vi "generateVang.vi"(5 "Vang_limit":dbl=4.0, 7 "PID Gains Angle":T1={"proportional gain (Kc)"=5.0, "integral time (Ti, min)"=0.0, "derivative time (Td, min)"=-2.0}, 8 "error in (no error)":errorcluster, 9 "Dest":dbl[](array[numeric])=[4500.0, 3000.0] format="%#_13g", 10 "Robot":refnum<class "Robot.lvclass">, 11 "Game in":refnum<class "Game.lvclass">) -> (0 "error out":errorcluster, 2 "Vang":dbl, 3 "Game out":refnum<class "Game.lvclass">)   [LabVIEW 2020, in "Game.lvclass"]
uses:
  Game.lvclass
  Robot_class/Robot.lvclass
  C:/RoboIME/SSL_AI/Object_class/Object.lvclass
  Object_class/Object.lvclass/Object.ctl
  Robot_class/Robot.lvclass/Robot.ctl
  <vilib>/Analysis/coordinate.llb/Wrap Angle (scalar).vi
  Object_class/Read x.vi
  Object_class/Read y.vi
  Robot_class/Read orientation.vi
  <vilib>/Analysis/NI_AAL_Angle.lvlib
panel:
  in  "Reinitialize":bool
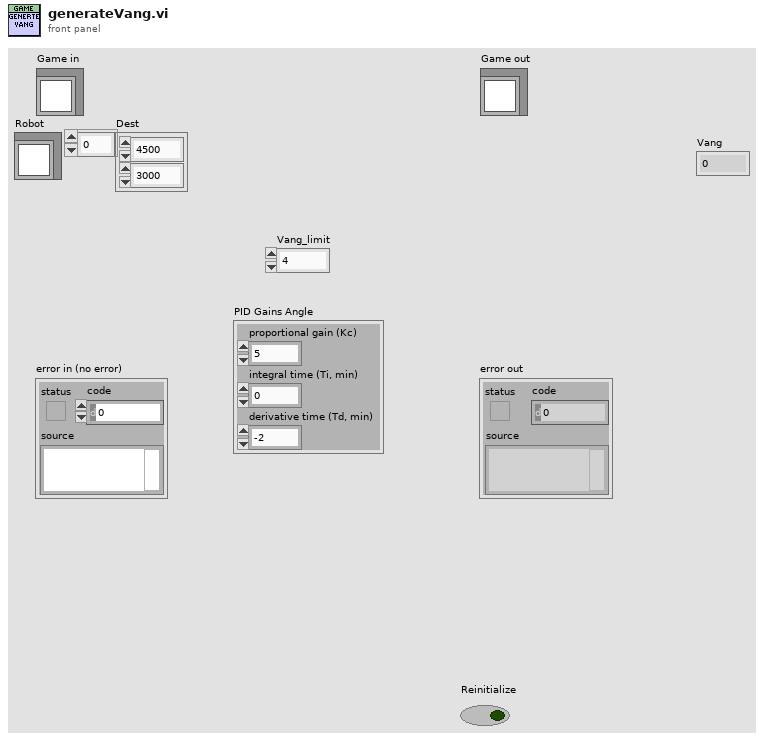
[diagram p1: front panel]
types:
  T1 = cluster{"proportional gain (Kc)":dbl, "integral time (Ti, min)":dbl, "derivative time (Td, min)":dbl}
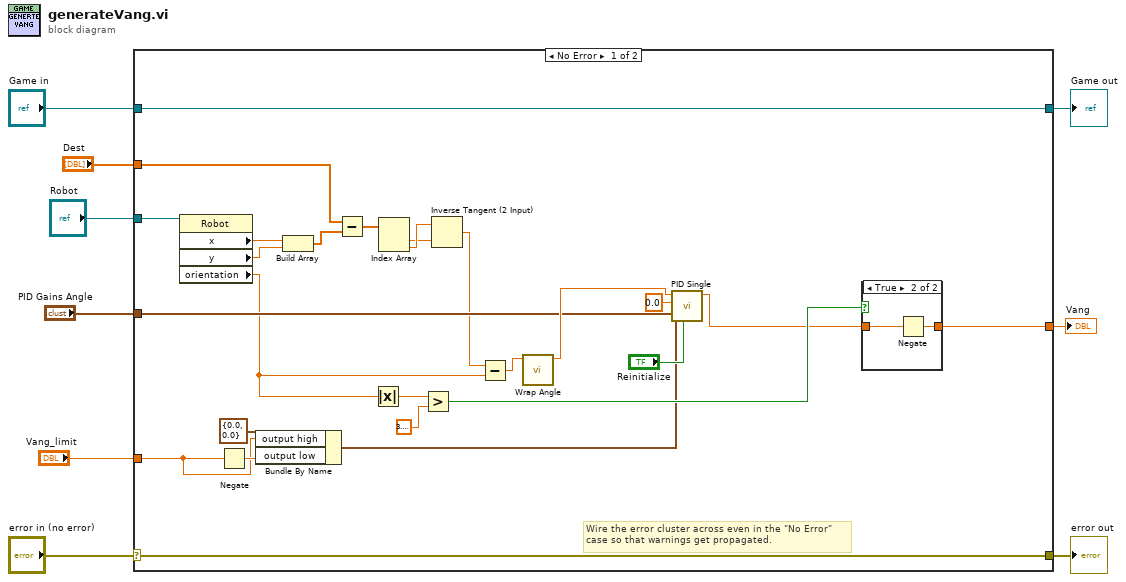
[diagram p0: block diagram]
diagram:
  n1 = case shown="No Error" "error in (no error)" {
    selector: "error in (no error)" -> [w34 w40]
    tunnel: [w34 w40] -> w8
    tunnel: [w35 w39] -> w6
    tunnel: "Game in" -> [w35 w39]
    tunnel: [w22 _] -> w5
    tunnel: "Vang_limit" -> [w21 _]
    tunnel: "PID Gains Angle" -> [w20 _]
    tunnel: "Robot" -> [w19 _]
    tunnel: "Dest" -> [w15 _]
    frame No Error {
      # "Wire the error cluster across even in the \"No Error\"\ncase so that warnings get propagated."
      n2 = property class="Robot"(reference=w19) -> ("x"=w17:dbl, "y"=w16:dbl, "orientation"=w18:dbl)  [unwired: 1 in, 2 out]
      n3 = Negate(x=w21) -> (-x=w24:dbl)
      n4 = Bundle By Name(cluster=cluster{"output high":dbl, "output low":dbl} {"output high"=0.0, "output low"=0.0}, "output high"=w21, "output low"=w24) -> (w23:cluster{"output high":dbl, "output low":dbl})
      n5 = Build Array(w17, w16) -> (w14:dbl[])
      n6 = Subtract(x=w15, y=w14) -> (x-y=w13:dbl[])
      n7 = Absolute Value(x=w18) -> (abs(x)=w33:dbl)
      n8 = Index Array(array=w13) -> (element #1=w11:dbl, element #2=w12:dbl)  [unwired: 2 in]
      n9 = Greater?(x=w33, y=3.141592653589793) -> (0:w32:bool)
      n10 = Inverse Tangent (2 Input)(1:w11, 2:w12) -> (0:w10:dbl)
      n11 = Subtract(x=w10, y=w18) -> (x-y=w30:dbl)
      n12 = call-poly <vilib>:"Wrap Angle.vi"("angle in"=w30) -> ("angle out"=w29:dbl)  [unwired: 9 in, 1 out]
      n13 = call "PID Single.vi"("initialize"="Reinitialize", "Limits"=w23, "PID gains in"=w20, "Variable"=0.0, "Setpoint"=w29) -> ("Out"=w26:dbl)  [unwired: 6 in]
      n14 = case shown="True" w32 {
        tunnel: w26 -> [w36 w38]
        tunnel: [w36 w37] -> w22
        frame False {
        }
        frame True {
          n15 = Negate(x=w38) -> (-x=w37:dbl)
        }
      }
    }
    frame Error {
    }
  }
  "error out" <- w8
  "Game out" <- w6
  "Vang" <- w5
